vi "Connect.vi"(8 "error in (no error)":errorcluster, 11 "Telnet V2 in":refnum<class "Telnet V2.lvclass">) -> (0 "error out":errorcluster, 3 "Telnet V2 out":refnum<class "Telnet V2.lvclass">)   [LabVIEW 2018, in "Telnet V2.lvlib" / "Telnet V2.lvclass"]
uses:
  Telnet V2.lvclass
  Telnet V2.lvclass/Telnet V2.ctl
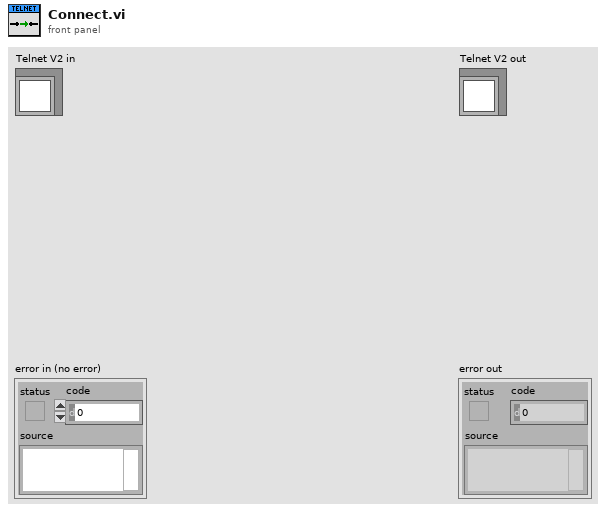
[diagram p1: front panel]
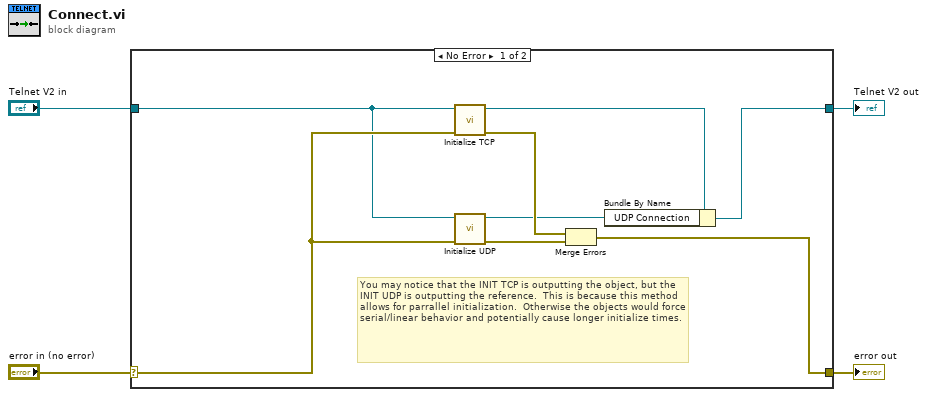
[diagram p0: block diagram]
diagram:
  n1 = case shown="No Error" "error in (no error)" {
    selector: "error in (no error)" -> [w10 w14]
    tunnel: [w11 w14] -> w3
    tunnel: [w7 w13] -> w1
    tunnel: "Telnet V2 in" -> [w6 w13]
    frame No Error {
      # "You may notice that the INIT TCP is outputting the object, but the INIT UDP is outputting the reference.  This is because this method allows for parrallel initialization.  Otherwise the objects would force serial/linear behavior and potentially cause longer initialize times."
      n2 = call "Initialize TCP.vi"("error in"=w10, "Telnet V2 in"=w6) -> ("error out"=w12:errorcluster, "Telnet V2 out"=w9:refnum<class "Telnet V2.lvclass">)  [unwired: 8 in]
      n3 = call "Initialize UDP.vi"("error in"=w10, "Telnet V2 in"=w6) -> ("error out"=w5:errorcluster, "connection ID"=w8:refnum<k16>)  [unwired: 8 in]
      n4 = Merge Errors(w12, w5) -> (w11:errorcluster)
      n5 = Bundle By Name(cluster=w9, "UDP Connection"=w8) -> (w7:refnum<class "Telnet V2.lvclass">)
    }
    frame Error {
    }
  }
  "error out" <- w3
  "Telnet V2 out" <- w1
